vi "RSZVB Select More Wave Quantities.vi"(5 "Wave Quantity Type (0: a)":i32(ring) items=["a", "b"], 6 "Source Port (1: Port 1)":i32=1, 7 "Wave Quantity Port Number (1)":i32=1, 8 "error in (no error)":errorcluster {"code" format="%.0x"}, 9 "Trace Name (Trc1)":string="Trc1", 10 "Channel (1)":i32=1, 11 "VISA session":refnum<visa-resource-name>) -> (0 "error out":errorcluster {"code" format="%.0x"}, 3 "dup VISA session":refnum<visa-resource-name>)   [LabVIEW 2011]
doc: "This VI select arbitrary wave quantities, e.g. for different detectors and source ports or more than 2 ports, frequency offsets, or mixed mode measurements.\n\nAssigns a measurement parameter to an existing trace or creates a trace and assigns a channel number, a name and a measurement parameter to it. The trace is not displayed.\n\nThe notation for wave quantities and the VIality of the More Wave Quantities is analogous to the definition of S-parameters.\n\nRemote-control command(s):\nCALCulate<Ch>:PARameter:SDEFine '<string>', 'A1D1' | 'B1D1' | 'B2D1' | 'A2D2' | 'B1D2' | 'B2D2' | ...\nCALCulate<Ch>:PARameter:MEASure '<string>', 'A1D1' | 'B1D1' | 'B2D1' | 'A2D2' | 'B1D2' | 'B2D2' | ..."
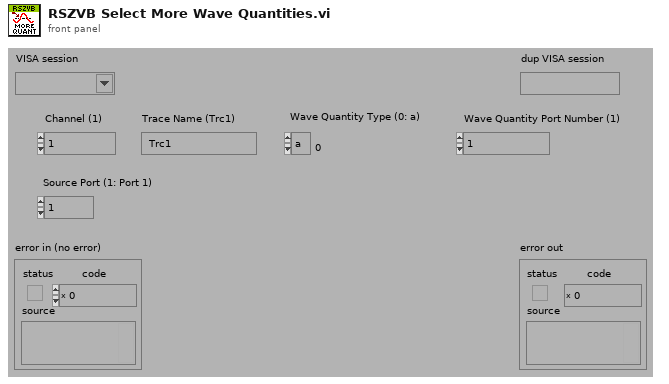
[diagram p1: front panel]
types:
  T1 = cluster{"Error Checking (T: On)":bool, "Installed Options":string[], "Data Valid?":bool, "Ports":i32, "Model":string[], "Option Checking (T: On)":bool}
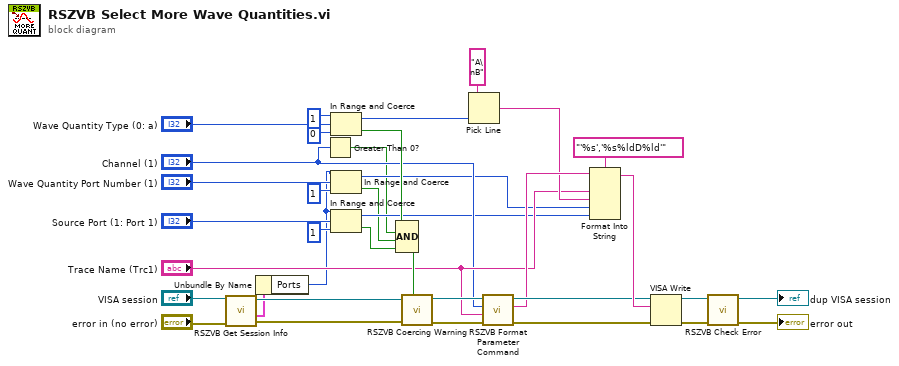
[diagram p0: block diagram]
diagram:
  n1 = call "RSZVB Get Session Info.vi"("error in (no error)"="error in (no error)", "VISA session"="VISA session") -> ("error out"=w3:errorcluster, "Session Info"=w2:T1, "dup VISA session"=w4:refnum<visa-resource-name>)  [unwired: 7 in]
  n2 = Unbundle By Name(w2) -> ("Ports"=w1:i32)
  n3 = Greater Than 0?(x="Channel (1)") -> (x > 0?=w9:bool)
  n4 = In Range and Coerce(upper limit=1, x="Wave Quantity Type (0: a)", lower limit=0) -> (coerced(x)=w24:i32, In Range?=w22:bool)
  n5 = In Range and Coerce(upper limit=w1, x="Wave Quantity Port Number (1)", lower limit=1) -> (coerced(x)=w11:i32, In Range?=w8:bool)
  n6 = In Range and Coerce(upper limit=w1, x="Source Port (1: Port 1)", lower limit=1) -> (coerced(x)=w10:i32, In Range?=w21:bool)
  n7 = Compound Arithmetic op=AND(w22, w9, w8, w21) -> (w32:bool)
  n8 = call "RSZVB Coercing Warning.vi"("In Range?"=w32, "error in (no error)"=w3, "VISA session"=w4) -> ("error out"=w29:errorcluster, "dup VISA session"=w28:refnum<visa-resource-name>)  [unwired: 7 in]
  n9 = Pick Line(multi-line string="A\nB", line index=w24) -> (output string=w23:string)  [unwired: 1 in]
  n10 = call "RSZVB Format Parameter Command.vi"("error in (no error)"=w29, "Trace Name (Trc1)"="Trace Name (Trc1)", "Channel (1)"="Channel (1)", "VISA session"=w28) -> ("error out"=w30:errorcluster, "Buffer"=w26:string, "dup VISA session"=w27:refnum<visa-resource-name>)  [unwired: 5 in]
  n11 = Format Into String(format string="'%s','%s%ldD%ld'", initial string=w26, "Trace Name (Trc1)", w23, w11, w10) -> (resulting string=w31:string)  [unwired: 1 in, 1 out]
  n12 = VISA Write(VISA resource name=w27, write buffer=w31, error in (no error)=w30) -> (VISA resource name out=w33:refnum<visa-resource-name>, error out=w34:errorcluster)  [unwired: 1 out]
  n13 = call "RSZVB Check Error.vi"("error in (no error)"=w34, "VISA session"=w33) -> ("error out"=→"error out":errorcluster, "dup VISA session"=→"dup VISA session":refnum<visa-resource-name>)  [unwired: 8 in]
